vi "Turn Only, Look at Both.vi"   [LabVIEW 2013]
uses:
  Team Code/Robot Global Data.vi
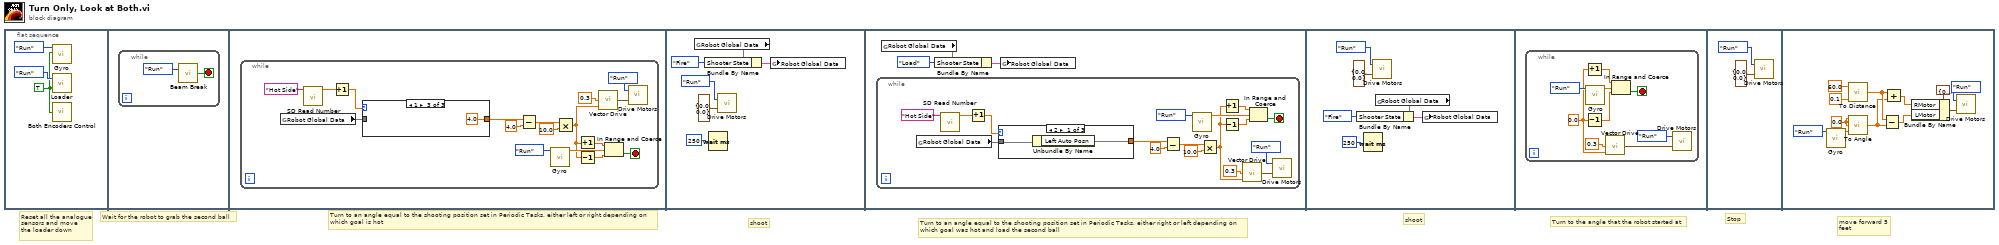
[diagram p0: block diagram]
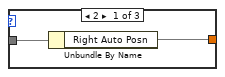
[diagram p2: hidden frame]
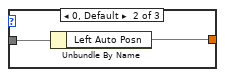
[diagram p3: hidden frame]
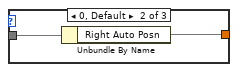
[diagram p4: hidden frame]
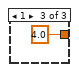
[diagram p5: hidden frame]
diagram:
  # "move forward 5\nfeet"
  # "Wait for the robot to grab the second ball"
  # "Stop"
  # "Turn to the angle that the robot started at"
  # "shoot"
  # "Turn to an angle equal to the shooting position set in Periodic Tasks, either right or left depending on\nwhich goal was hot and load the second ball"
  # "shoot"
  # "Turn to an angle equal to the shooting position set in Periodic Tasks, either left or right depending on\nwhich goal is hot"
  # "Reset all the analogue\nsensors and move \nthe loader down"
  n1 = flat-sequence {
    frame #0 {
      w1 = TRUE ("Reset")
      n2 = call "Gyro.vi"("Reset"=w1, "Enum"=enum16{"Start", "Run", "End"}."Run") -> ()  [unwired: 9 in, 1 out]
      n3 = call "Loader.vi"("Down (Forward)"=w1, "Enum"=enum16{"Start", "Run", "End"}."Run") -> ()  [unwired: 1 out]
      n4 = call "Both Encoders Control.vi"("Reset Both"=w1) -> ()  [unwired: 2 out]
    }
    frame #1 {
      n5 = while {
        stop <- w4 stop-if-true
        n6 = call "Beam Break.vi"("Enum"=enum16{"Start", "Run", "End"}."Run") -> ("Broken"=w4:bool)  [unwired: 1 in]
      }
    }
    frame #2 {
      n7 = while {
        stop <- w18 stop-if-true
        n8 = global read "Robot Global Data.vi" "Robot Global Data"() -> (w13)
        n9 = call <vilib>:"SD Read Number.vi"("Name"="Hot Side") -> ("Numeric"=w8:dbl)  [unwired: 8 in, 2 out]
        n10 = Increment(x=w8) -> (x+1=w6:dbl)
        n11 = case shown="1" w6 {
          tunnel: w13 -> [w24 w26 _]
          tunnel: [w23 w25 4.0 ("y")] -> w7
          frame 2 {
            n12 = Unbundle By Name(w24) -> ("Right Auto Posn"=w23)
          }
          frame 0, Default {
            n13 = Unbundle By Name(w26) -> ("Left Auto Posn"=w25)
          }
          frame 1 {
          }
        }
        n14 = Subtract(x=w7, y=4.0) -> (x-y=w10:dbl)
        n15 = call "Gyro.vi"("Enum"=enum16{"Start", "Run", "End"}."Run") -> ("Angle"=w19:dbl)  [unwired: 10 in]
        n16 = Multiply(x=w10, y=10.0) -> (x*y=w15:dbl)
        n17 = Increment(x=w15) -> (x+1=w16:dbl)
        n18 = Decrement(x=w15) -> (x-1=w14:dbl)
        n19 = call "Vector Drive.vi"("Angle"=w15, "Min. Power"=0.3) -> ("Motor Powers"=w22:cluster{"RMotor":dbl, "LMotor":dbl})  [unwired: 1 in]
        n20 = In Range and Coerce(upper limit=w16, x=w19, lower limit=w14) -> (In Range?=w18:bool)  [unwired: 1 out]
        n21 = call "Drive Motors.vi"("Motor Powers"=w22, "Enum"=enum16{"Start", "Run", "End"}."Run") -> ()
      }
    }
    frame #3 {
      n22 = global read "Robot Global Data.vi" "Robot Global Data"() -> (w28)
      n23 = Bundle By Name(cluster=w28, "Shooter State"=enum16{"Nothing", "Fire", "Load"}."Fire") -> (w29:cluster{})
      n24 = Wait (ms)(milliseconds to wait=u32 250) -> ()  [unwired: 1 out]
      n25 = call "Drive Motors.vi"("Motor Powers"=cluster{"RMotor":dbl, "LMotor":dbl} {"RMotor"=0.0, "LMotor"=0.0}, "Enum"=enum16{"Start", "Run", "End"}."Run") -> ()
      n26 = global write "Robot Global Data.vi" "Robot Global Data"(w29) -> ()
    }
    frame #4 {
      n27 = while {
        stop <- w49 stop-if-true
        n28 = global read "Robot Global Data.vi" "Robot Global Data"() -> (w41)
        n29 = call <vilib>:"SD Read Number.vi"("Name"="Hot Side") -> ("Numeric"=w39:dbl)  [unwired: 8 in, 2 out]
        n30 = Increment(x=w39) -> (x+1=w37:dbl)
        n31 = case shown="2" w37 {
          tunnel: w41 -> [w55 w57 _]
          tunnel: [w54 w56 4.0 ("y")] -> w40
          frame 2 {
            n32 = Unbundle By Name(w55) -> ("Left Auto Posn"=w54)
          }
          frame 0, Default {
            n33 = Unbundle By Name(w57) -> ("Right Auto Posn"=w56)
          }
          frame 1 {
          }
        }
        n34 = Subtract(x=w40, y=4.0) -> (x-y=w45:dbl)
        n35 = call "Gyro.vi"("Enum"=enum16{"Start", "Run", "End"}."Run") -> ("Angle"=w50:dbl)  [unwired: 10 in]
        n36 = Multiply(x=w45, y=10.0) -> (x*y=w42:dbl)
        n37 = Increment(x=w42) -> (x+1=w47:dbl)
        n38 = Decrement(x=w42) -> (x-1=w46:dbl)
        n39 = call "Vector Drive.vi"("Angle"=w42, "Min. Power"=0.3 ("Power")) -> ("Motor Powers"=w53:cluster{"RMotor":dbl, "LMotor":dbl})  [unwired: 1 in]
        n40 = In Range and Coerce(upper limit=w47, x=w50, lower limit=w46) -> (In Range?=w49:bool)  [unwired: 1 out]
        n41 = call "Drive Motors.vi"("Motor Powers"=w53, "Enum"=enum16{"Start", "Run", "End"}."Run") -> ()
      }
      n42 = global read "Robot Global Data.vi" "Robot Global Data"() -> (w35)
      n43 = Bundle By Name(cluster=w35, "Shooter State"=enum16{"Nothing", "Fire", "Load"}."Load") -> (w34:cluster{})
      n44 = global write "Robot Global Data.vi" "Robot Global Data"(w34) -> ()
    }
    frame #5 {
      n45 = Wait (ms)(milliseconds to wait=u32 250) -> ()  [unwired: 1 out]
      n46 = call "Drive Motors.vi"("Motor Powers"=cluster{"RMotor":dbl, "LMotor":dbl} {"RMotor"=0.0, "LMotor"=0.0}, "Enum"=enum16{"Start", "Run", "End"}."Run") -> ()
      n47 = global read "Robot Global Data.vi" "Robot Global Data"() -> (w60)
      n48 = Bundle By Name(cluster=w60, "Shooter State"=enum16{"Nothing", "Fire", "Load"}."Fire") -> (w59:cluster{})
      n49 = global write "Robot Global Data.vi" "Robot Global Data"(w59) -> ()
    }
    frame #6 {
      n50 = while {
        stop <- w69 stop-if-true
        w66 = 0.0 ("x")
        n51 = Increment(x=w66) -> (x+1=w68:dbl)
        n52 = Decrement(x=w66) -> (x-1=w67:dbl)
        n53 = call "Gyro.vi"("Enum"=enum16{"Start", "Run", "End"}."Run") -> ("Angle"=w70:dbl)  [unwired: 10 in]
        n54 = call "Vector Drive.vi"("Angle"=w66, "Min. Power"=0.3) -> ("Motor Powers"=w73:cluster{"RMotor":dbl, "LMotor":dbl})  [unwired: 1 in]
        n55 = In Range and Coerce(upper limit=w68, x=w70, lower limit=w67) -> (In Range?=w69:bool)  [unwired: 1 out]
        n56 = call "Drive Motors.vi"("Motor Powers"=w73, "Enum"=enum16{"Start", "Run", "End"}."Run") -> ()
      }
    }
    frame #7 {
      n57 = call "Drive Motors.vi"("Motor Powers"=cluster{"RMotor":dbl, "LMotor":dbl} {"RMotor"=0.0, "LMotor"=0.0}, "Enum"=enum16{"Start", "Run", "End"}."Run") -> ()
    }
    frame #8 {
      w82 = 0.0 ("Min. Power")
      n58 = call "Gyro.vi"("Enum"=enum16{"Start", "Run", "End"}."Run") -> ("Angle"=w83:dbl)  [unwired: 10 in]
      n59 = call "To Distance.vi"("Min. Power"=0.1, "Destination Dist (in)"=60.0 ("Destination Dist")) -> ("Base Speed"=w81:dbl)  [unwired: 1 in]
      n60 = call "To Angle.vi"("Current Angle"=w83, "Min. Power"=w82, "Destination Angle"=w82) -> ("Power Change"=w80:dbl)
      n61 = Subtract(x=w81, y=w80) -> (x-y=w79:dbl)
      n62 = Add(x=w81, y=w80) -> (x+y=w78:dbl)
      n63 = Bundle By Name(cluster=cluster{"RMotor":dbl, "LMotor":dbl} {"RMotor"=0.0, "LMotor"=0.0} ("Motor Powers"), "RMotor"=w78, "LMotor"=w79) -> (w76:cluster{"RMotor":dbl, "LMotor":dbl})
      n64 = call "Drive Motors.vi"("Motor Powers"=w76, "Enum"=enum16{"Start", "Run", "End"}."Run") -> ()
    }
  }
